vi "GetAllDeviceParameterNames.vi"(8 "error in":errorcluster, 10 "Device Command":string, 11 "connection ID in":refnum<k5>) -> (0 "error out":errorcluster, 1 "Error Info":T1, 2 "Device Parameter Names":string[](array[string]), 3 "connection ID out":refnum<k5>, 4 "log string":string, 5 "OK":bool)   [LabVIEW 2020, in "ProdigyRemoteControl.lvlib"]
uses:
  ProdigyRemoteControl.lvlib
  DEFINITIONS/DEF_RcError.ctl
  DEFINITIONS/DEF_RcCmd.ctl
  <vilib>/regexp/Match Regular Expression.xnode
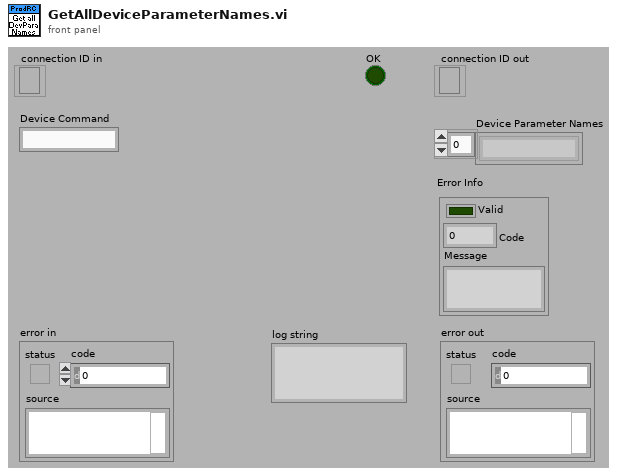
[diagram p1: front panel]
types:
  T1 = typedef "ProdigyRemoteControl.lvlib/DEF_RcError.ctl" = cluster{"Valid":bool, "Code":u16, "Message":string}
  T2 = typedef "ProdigyRemoteControl.lvlib/DEF_RcCmd.ctl" = string
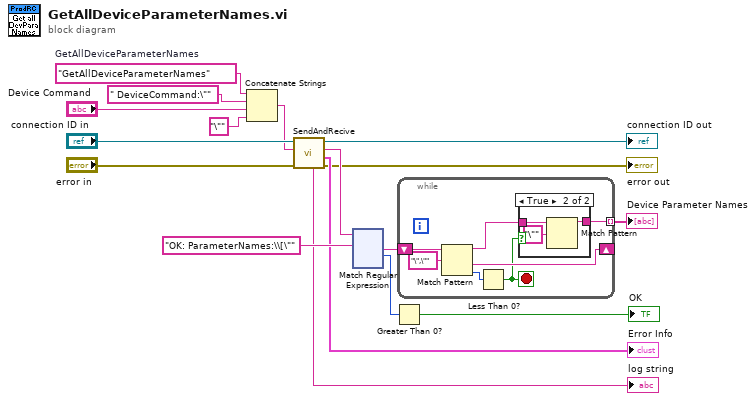
[diagram p0: block diagram]
diagram:
  w5 = T2 "GetAllDeviceParameterNames"  # GetAllDeviceParameterNames
  n1 = Concatenate Strings(w5, " DeviceCommand:\"" ("string"), "Device Command", "\"" ("string")) -> (w1:string)
  n2 = call "SendAndRecive.vi"("error in"="error in", "Command"=w1, "connection ID in"="connection ID in") -> ("error out"=→"error out":errorcluster, "Error Info"=→"Error Info":T1, "Answer"=w15:string, "connection ID out"=→"connection ID out":refnum<k5>, "Log String"=→"log string":string)  [unwired: 4 in]
  n3 = xnode "Match Regular Expression"("input string"=w15, "regular expression"="OK: ParameterNames:\\[\"") -> ("after match"=w14:string, "offset past match"=w7:i32)  [unwired: 4 in, 3 out]
  n4 = Greater Than 0?(x=w7) -> (x > 0?=→"OK":bool)
  n5 = while {
    shift-right: [w21] -> _
    shift-left: w14 -> [w24]
    tunnel: [w19] -> w17 mode=indexing
    stop <- w18 stop-if-true
    n6 = Match Pattern(string=w24, regular expression="\",\"") -> (before substring=w20:string, after substring=w21:string, offset past match=w22:i32)  [unwired: 1 in, 1 out]
    n7 = Less Than 0?(x=w22) -> (x < 0?=w18:bool)
    n8 = case shown="True" w18 {
      tunnel: w20 -> [w25 w28]
      tunnel: [w25 w27] -> w19
      frame False {
      }
      frame True {
        n9 = Match Pattern(string=w28, regular expression="\"") -> (before substring=w27:string)  [unwired: 1 in, 3 out]
      }
    }
  }
  "Device Parameter Names" <- w17
